vi "shutter_new.vi"(1 "error in":errorcluster, 2 "ShutterID":i32 min=0 max=65535, 3 "Shutter Position":bool, 4 "ObjectPtr":i32) -> (0 "error out":errorcluster)   [LabVIEW 2014]
panel:
  out "Status":string
  out "Numeric":i32=153
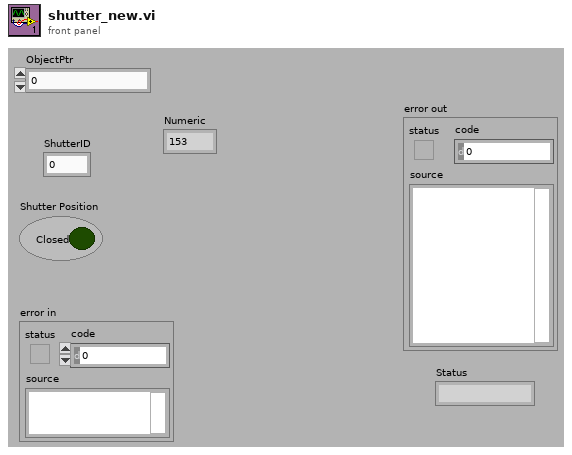
[diagram p1: front panel]
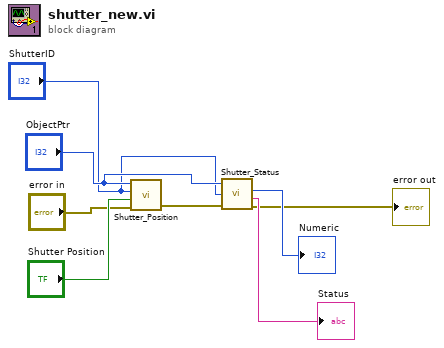
[diagram p0: block diagram]
diagram:
  n1 = call "Shutter_Position.vi"("error in"="error in", "Shutter Position"="Shutter Position", "ShutterID"="ShutterID", "ObjectPtr"="ObjectPtr") -> ("error out"=w8:errorcluster)  [unwired: 2 in]
  n2 = call "Shutter_Status.vi"("ObjectPtr"="ObjectPtr", "ShutterID"="ShutterID", "error in"=w8) -> ("Position"=→"Numeric":i32, "Status"=→"Status":string, "error out"=→"error out":errorcluster)  [unwired: 1 out]
